vi "QMH Simple Clock Example.vi"() -> ()   [LabVIEW 2013]
uses:
  <userlib>/QMH/examples/Simple Clock/QMH Simple Clock Style.ctl
  <userlib>/QMH/QMH Add Message to Queue (Single Element).vi
  <userlib>/QMH/QMH Add Message to Queue (Array).vi
  <vilib>/Utility/config.llb/Read Key (I32).vi
  <vilib>/Utility/config.llb/Write Key (I32).vi
  <vilib>/Utility/config.llb/NI_LVConfig.lvlib
panel:
  in  "Save State":bool
  out "Seconds":bool[](array[boolean])
  out "Seconds Tens":bool[](array[boolean])
  out "Minutes":bool[](array[boolean])
  out "Minutes Tens":bool[](array[boolean])
  out "Hours":bool[](array[boolean])
  out "Hours Tens":bool[](array[boolean])
  out "Digital":string
  in  "Clock Style":T1
  out "Hour":dbl(knob) scale=0.0..12.0
  out "Minute":dbl(knob) scale=0.0..12.0 scale format="%#.0f"
  out "Status":string
  in  "About":bool
  in  "Exit":bool
  in  "State Variables":cluster{"Config File":path, "Clock Style":T1}
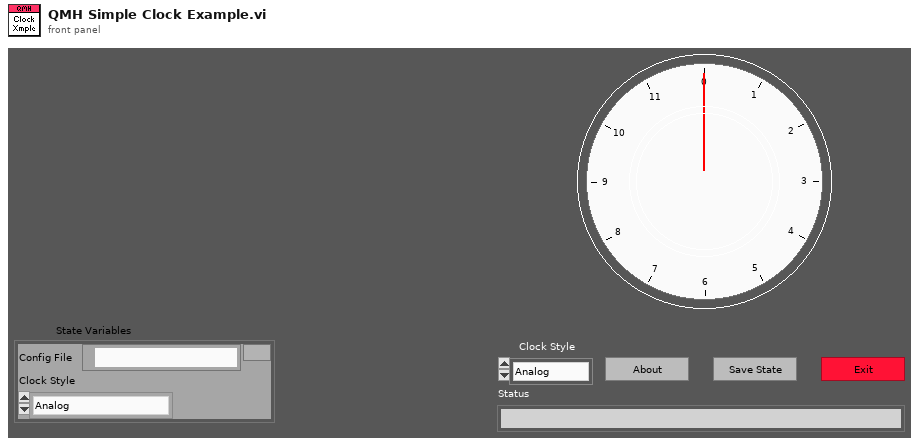
[diagram p1: front panel]
types:
  T1 = typedef "QMH Simple Clock Style.ctl" = enum16{"Analog", "Digital", "Binary"}
  T2 = typedef "LVDateTimeRec.ctl" = cluster{"fractional second":dbl, "second":i32, "minute":i32, "hour":i32, "day of month":i32, "month":i32, "year":i32, "day of week":i32, "day of year":i32, "DST":i32}
  T3 = typedef "NI_LVConfig.lvlib/Config Data RefNum.ctl" = refnum<k1>
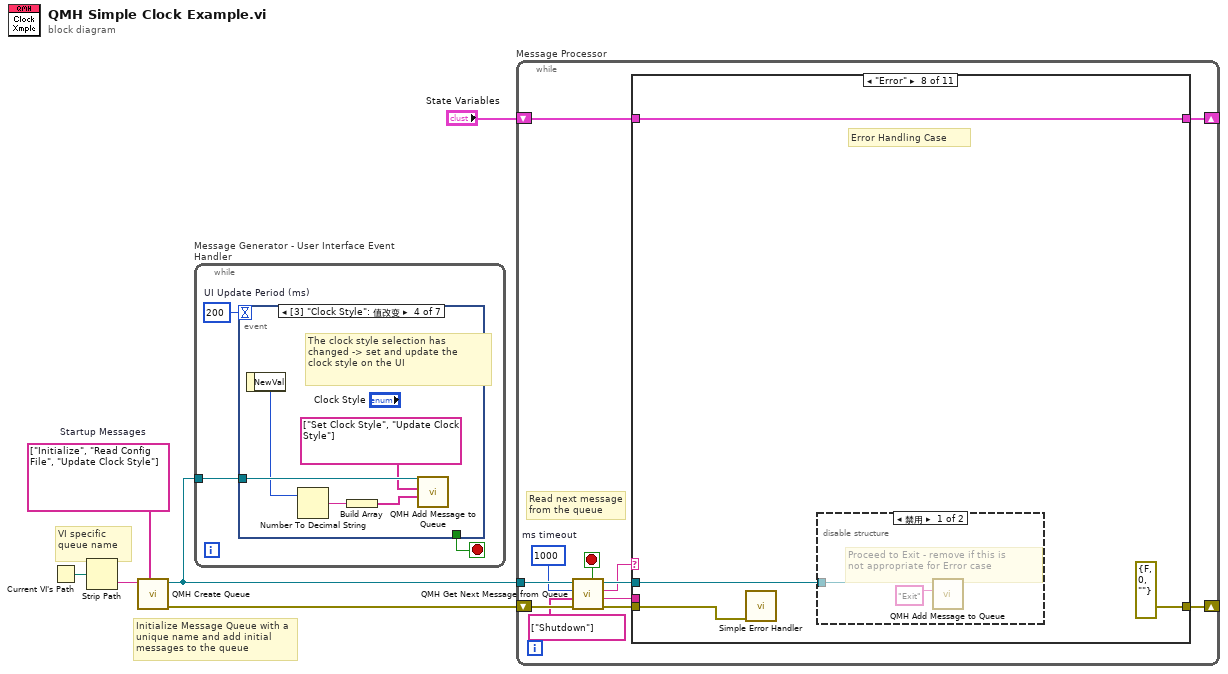
[diagram p0: block diagram]
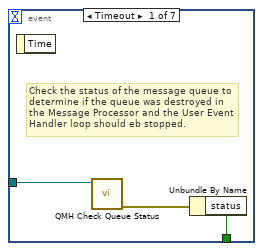
[diagram p2: hidden frame]
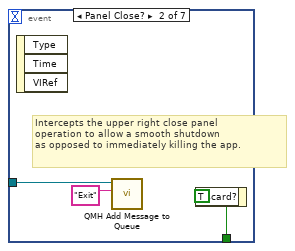
[diagram p3: hidden frame]
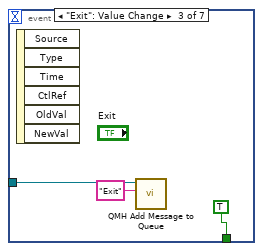
[diagram p4: hidden frame]
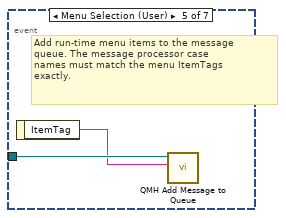
[diagram p5: hidden frame]
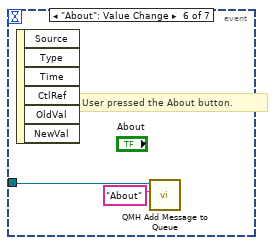
[diagram p6: hidden frame]
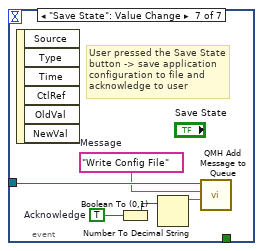
[diagram p7: hidden frame]
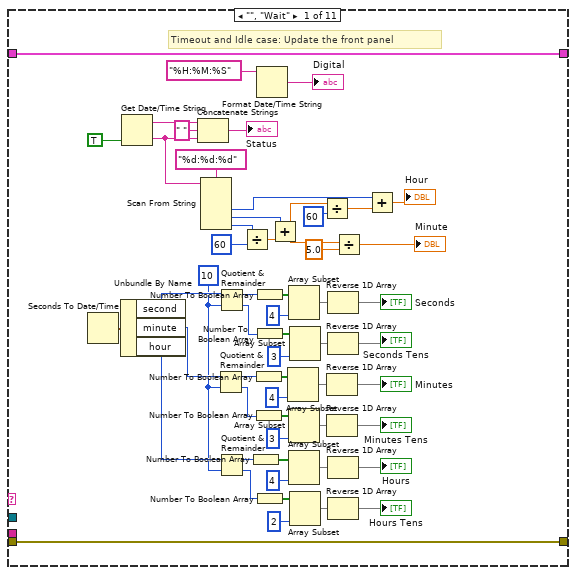
[diagram p8: hidden frame]
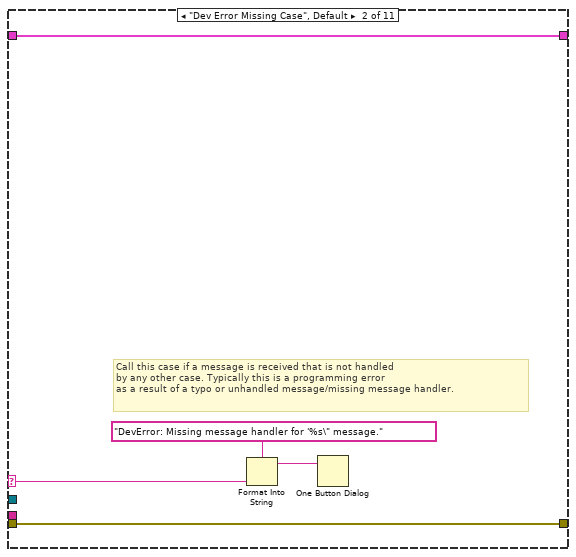
[diagram p9: hidden frame]
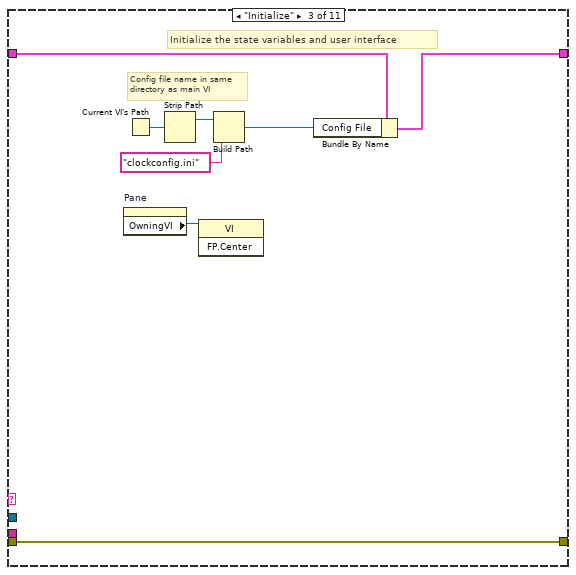
[diagram p10: hidden frame]
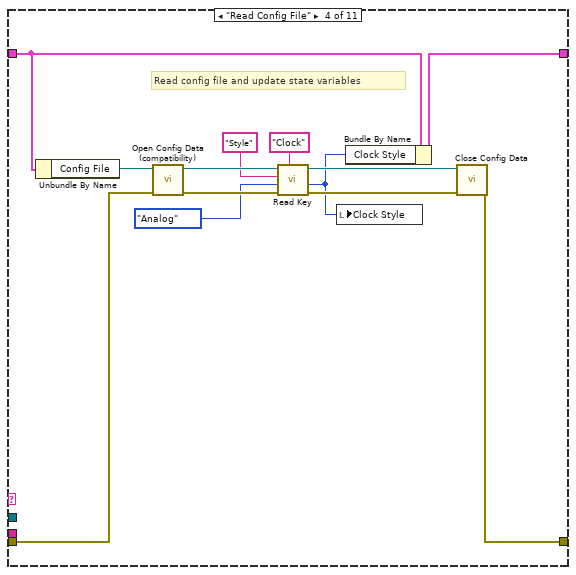
[diagram p11: hidden frame]
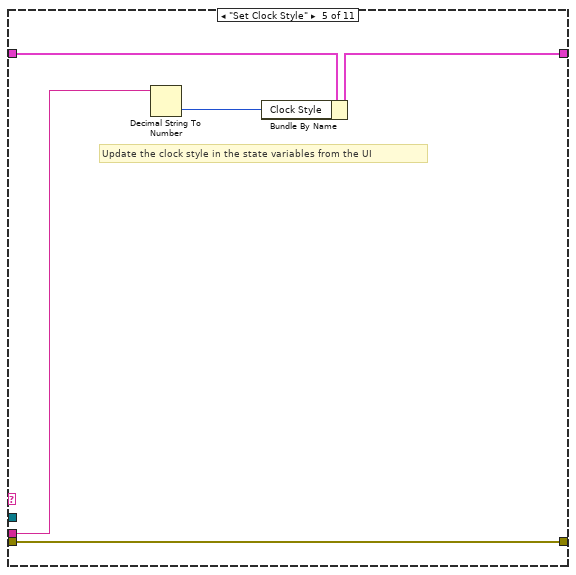
[diagram p12: hidden frame]
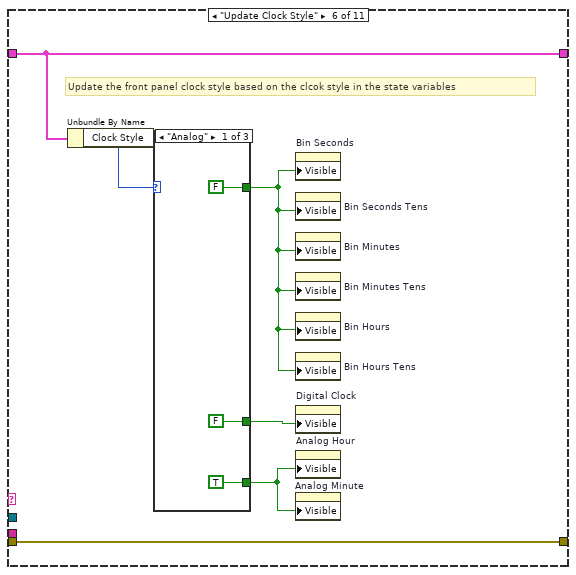
[diagram p13: hidden frame]
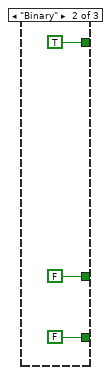
[diagram p14: hidden frame]
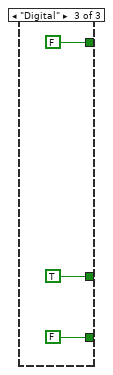
[diagram p15: hidden frame]
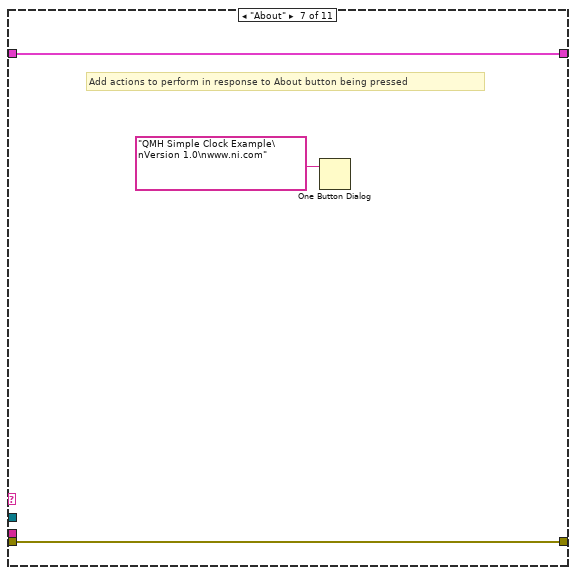
[diagram p16: hidden frame]
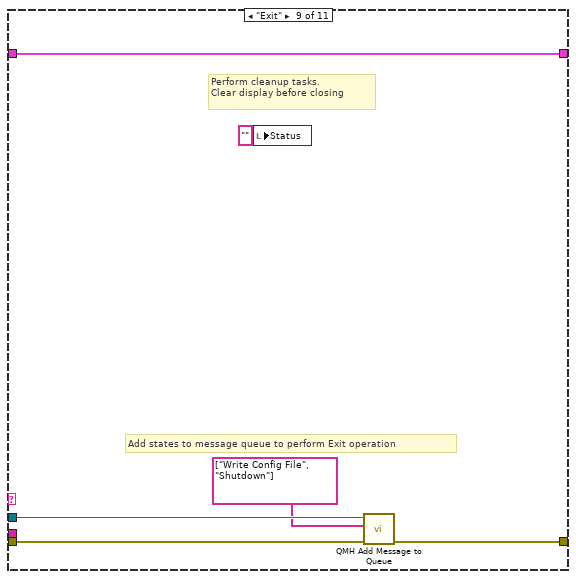
[diagram p18: hidden frame]
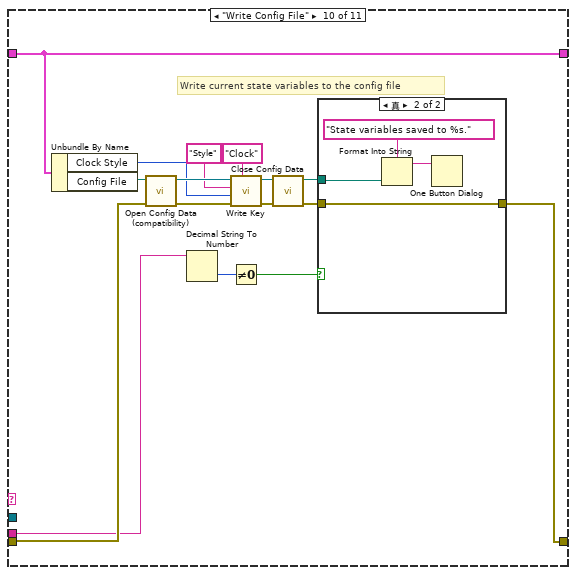
[diagram p19: hidden frame]
diagram:
  w5 = string[] ["Initialize", "Read Config File", "Update Clock Style"]  # Startup Messages
  # "VI specific\nqueue name"
  # "Initialize Message Queue with a unique name and add initial messages to the queue"
  n1 = Current VI's Path() -> (path=w2:path)
  n2 = Strip Path(path=w2) -> (name=w1:string)  [unwired: 1 out]
  n3 = call <userlib>:"QMH Create Queue.vi"("Initial Messages"=w5, "Message queue name (unnamed)"=w1) -> ("error out"=w6:errorcluster, "queue out"=w3:refnum<queue>)  [unwired: 8 in]
  n4 = while "Message Generator - User Interface Event Handler" {
    tunnel: w3 -> [w7]
    stop <- w8 stop-if-true
    w9 = 200  # UI Update Period (ms)
    n5 = event shown="[3] \"Clock Style\": 值改变" {
      selector: _ -> [_ _ _ _ _ _ _]
      dyn-events: _ -> [_ _ _ _ _ _ _]
      timeout: w9 -> [_ _ _ _ _ _ _]
      tunnel: [w12 w15 TRUE ("Discard?") _ _ _ _] -> w8
      tunnel: w7 -> [w11 w14 w17 w23 w25 w27 w32]
      event Timeout {
        # "Check the status of the message queue to determine if the queue was destroyed in the Message Processor and the User Event Handler loop should eb stopped."
        n6 = event-data() -> ()  [unwired: 1 in, 1 out]
        n7 = call <userlib>:"QMH Check Queue Status.vi"("queue in"=w11) -> ("error out"=w10:errorcluster)  [unwired: 7 in, 2 out]
        n8 = Unbundle By Name(w10) -> ("status"=w12:bool)
      }
      event Panel Close? {
        w15 = TRUE ("Discard?")
        # "Intercepts the upper right close panel\noperation to allow a smooth shutdown\nas opposed to immediately killing the app."
        n9 = event-data() -> ()  [unwired: 1 in, 3 out]
        n10 = call-poly <userlib>:"QMH Add Message to Queue.vi"("Message"="Exit", "queue in"=w14) -> ()  [unwired: 8 in, 2 out]
        n11 = event-data("Discard?"=w15) -> ()  [unwired: 1 in, 1 out]
      }
      event "Exit": Value Change {
        n12 = event-data() -> ()  [unwired: 1 in, 6 out]
        n13 = call-poly <userlib>:"QMH Add Message to Queue.vi"("Message"="Exit", "queue in"=w17) -> ()  [unwired: 8 in, 2 out]
      }
      event Value Change {
        # "The clock style selection has\nchanged -> set and update the\nclock style on the UI"
        n14 = event-data() -> ("NewVal"=w19:T1)  [unwired: 1 in]
        n15 = Number To Decimal String(number=w19) -> (decimal integer string=w21:string)  [unwired: 1 in]
        n16 = Build Array(w21) -> (w20:string[])
        n17 = call-poly <userlib>:"QMH Add Message to Queue.vi"("Parameters"=w20, "Messages"=string[] ["Set Clock Style", "Update Clock Style"], "queue in"=w23) -> ()  [unwired: 7 in, 2 out]
      }
      event Menu Selection (User) {
        # "Add run-time menu items to the message\nqueue. The message processor case\nnames must match the menu ItemTags\nexactly."
        n18 = event-data() -> ("ItemTag"=w24:string)  [unwired: 1 in]
        n19 = call-poly <userlib>:"QMH Add Message to Queue.vi"("Message"=w24, "queue in"=w25) -> ()  [unwired: 8 in, 2 out]
      }
      event "About": Value Change {
        # "User pressed the About button."
        n20 = event-data() -> ()  [unwired: 1 in, 6 out]
        n21 = call-poly <userlib>:"QMH Add Message to Queue.vi"("Message"="About", "queue in"=w27) -> ()  [unwired: 8 in, 2 out]
      }
      event "Save State": Value Change {
        w30 = TRUE  # Acknowledge
        w31 = "Write Config File"  # Message
        # "User pressed the Save State button -> save application configuration to file and acknowledge to user"
        n22 = event-data() -> ()  [unwired: 1 in, 6 out]
        n23 = Boolean To (0,1)(Boolean=w30) -> (0, 1=w28:i16)
        n24 = Number To Decimal String(number=w28) -> (decimal integer string=w29:string)  [unwired: 1 in]
        n25 = call-poly <userlib>:"QMH Add Message to Queue.vi"("Parameter"=w29, "Message"=w31, "queue in"=w32) -> ()  [unwired: 7 in, 2 out]
      }
    }
  }
  n26 = while "Message Processor" {
    shift-left: w6 -> [w38]
    shift-right: [w39] -> _
    tunnel: w3 -> [w37]
    shift-left: "State Variables" -> [w44]
    shift-right: [w43] -> _
    stop <- w42 stop-if-true
    w35 = 1000  # ms timeout
    # "Read next message from the queue"
    n27 = call <userlib>:"QMH Get Next Message from Queue.vi"("error in (no error)"=w38, "Termination List ([Exit])"=string[] ["Shutdown"], "ms timeout (1)"=w35, "queue in"=w37) -> ("error out"=w40:errorcluster, "Next Parameter"=w34:string, "Next Message"=w36:string, "queue out"=w41:refnum<queue>, "Stop QMH"=w42:bool)  [unwired: 2 in]
    n28 = case shown="\"Error\"" w36 {
      selector: w36 -> [_ w103 _ _ _ _ _ _ _ _ _]
      tunnel: [w100 w105 w111 w122 w129 w136 w148 w153 w161 w169 w184] -> w43
      tunnel: w44 -> [w100 w105 w112 w118 w130 w136 w148 w153 w161 w169 w184]
      tunnel: w41 -> [_ _ _ _ _ _ _ w150 w159 _ w185]
      tunnel: w40 -> [w99 w104 w113 w116 w131 w137 w149 w151 w158 w168 w186]
      tunnel: [w99 w104 w113 w115 w131 w137 w149 errorcluster {"status"=FALSE, "code"=0, "source"=""} ("error out") w157 w162 w183] -> w39
      tunnel: w34 -> [_ _ _ _ w128 _ _ _ _ w167 _]
      frame "", "Wait" {
        w56 = 10 ("y")
        # "Timeout and Idle case: Update the front panel"
        n29 = Seconds To Date/Time() -> (date time rec=w82:T2)  [unwired: 2 in]
        n30 = Unbundle By Name(w82) -> ("second"=w81:i32, "minute"=w58:i32, "hour"=w57:i32)
        n31 = Get Date/Time String(want seconds? (F)=TRUE) -> (date string=w98:string, time string=w47:string)  [unwired: 2 in]
        n32 = Concatenate Strings(w98, " " ("string"), w47) -> (→"Status":string)
        n33 = Scan From String(format string="%d:%d:%d", input string=w47) -> (output 1=w88:i32, output 2=w91:i32, output 3=w83:i32)  [unwired: 5 in, 3 out]
        n34 = Quotient & Remainder(x=w58, y=w56) -> (x-y*floor(x/y)=w49:i32, floor(x/y)=w65:i32)
        n35 = Quotient & Remainder(x=w81, y=w56) -> (x-y*floor(x/y)=w80:i32, floor(x/y)=w79:i32)
        n36 = Quotient & Remainder(x=w57, y=w56) -> (x-y*floor(x/y)=w54:i32, floor(x/y)=w64:i32)
        n37 = Divide(x=w83, y=60) -> (x/y=w92:dbl)
        n38 = Number To Boolean Array(number=w54) -> (Boolean array=w53:bool[])
        n39 = Number To Boolean Array(number=w49) -> (Boolean array=w48:bool[])
        n40 = Number To Boolean Array(number=w65) -> (Boolean array=w69:bool[])
        n41 = Number To Boolean Array(number=w80) -> (Boolean array=w77:bool[])
        n42 = Number To Boolean Array(number=w79) -> (Boolean array=w74:bool[])
        n43 = Number To Boolean Array(number=w64) -> (Boolean array=w60:bool[])
        n44 = Format Date/Time String(time format string (%c)="%H:%M:%S") -> (date/time string=→"Digital":string)  [unwired: 2 in]
        n45 = Add(x=w91, y=w92) -> (x+y=w86:dbl)
        n46 = Array Subset(array=w48, length=4) -> (w66:bool[])  [unwired: 1 in]
        n47 = Array Subset(array=w77, length=4) -> (w78:bool[])  [unwired: 1 in]
        n48 = Array Subset(array=w69, length=3) -> (w70:bool[])  [unwired: 1 in]
        n49 = Array Subset(array=w53, length=4) -> (w63:bool[])  [unwired: 1 in]
        n50 = Array Subset(array=w74, length=3) -> (w73:bool[])  [unwired: 1 in]
        n51 = Array Subset(array=w60, length=2) -> (w59:bool[])  [unwired: 1 in]
        n52 = Divide(x=w86, y=60) -> (x/y=w89:dbl)
        n53 = Reverse 1D Array(array=w66) -> (reversed array=→"Minutes":bool[])
        n54 = Reverse 1D Array(array=w70) -> (reversed array=→"Minutes Tens":bool[])
        n55 = Reverse 1D Array(array=w78) -> (reversed array=→"Seconds":bool[])
        n56 = Reverse 1D Array(array=w73) -> (reversed array=→"Seconds Tens":bool[])
        n57 = Reverse 1D Array(array=w63) -> (reversed array=→"Hours":bool[])
        n58 = Reverse 1D Array(array=w59) -> (reversed array=→"Hours Tens":bool[])
        n59 = Divide(x=w86, y=5.0) -> (x/y=→"Minute":dbl)
        n60 = Add(x=w88, y=w89) -> (x+y=→"Hour":dbl)
      }
      frame "Dev Error Missing Case", Default {
        # "Call this case if a message is received that is not handled \nby any other case. Typically this is a programming error\nas a result of a typo or unhandled message/missing message handler."
        n61 = Format Into String(format string="DevError: Missing message handler for '%s\" message." ("message"), w103) -> (resulting string=w101:string)  [unwired: 2 in, 1 out]
        n62 = One Button Dialog(message=w101) -> ()  [unwired: 1 in, 1 out]
      }
      frame "Initialize" {
        # "Config file name in same directory as main VI"
        # "Initialize the state variables and user interface"
        n63 = property on="Pane" class="Pane"() -> ("OwningVI"=w106:refnum<vi>)  [unwired: 2 in, 2 out]
        n64 = Current VI's Path() -> (path=w110:path)
        n65 = Strip Path(path=w110) -> (stripped path=w109:path)  [unwired: 1 out]
        n66 = invoke class="VI" method="FP.Center"(reference=w106) -> ()  [unwired: 2 in, 3 out]
        n67 = Build Path(base path=w109, name or relative path="clockconfig.ini") -> (appended path=w107:path)
        n68 = Bundle By Name(cluster=w112, "Config File"=w107) -> (w111:cluster{"Config File":path, "Clock Style":T1})
      }
      frame "Read Config File" {
        # "Read config file and update state variables"
        n69 = Unbundle By Name(w118) -> ("Config File"=w117:path)
        n70 = call <vilib>:"Open Config Data (compatibility).vi"("error in (no error)"=w116, "configuration file path"=w117) -> ("error out"=w126:errorcluster, "refnum"=w125:T3)  [unwired: 7 in, 1 out]
        n71 = call-poly <vilib>:"Read Key.vi"("section"="Clock", "error in (no error)"=w126, "default value"=QMH_Simple_Clock_Style."Analog" ("NewVal"), "key"="Style", "refnum"=w125) -> ("error out"=w119:errorcluster, "value"=w114:i32, "refnum out"=w120:T3)  [unwired: 3 in, 1 out]
        n72 = local write "Clock Style"(w114) -> ()
        n73 = Bundle By Name(cluster=w118, "Clock Style"=w114) -> (w122:cluster{"Config File":path, "Clock Style":T1})
        n74 = call <vilib>:"Close Config Data.vi"("error in (no error)"=w119, "refnum"=w120) -> ("error out"=w115:errorcluster)  [unwired: 8 in, 1 out]
      }
      frame "Set Clock Style" {
        # "Update the clock style in the state variables from the UI"
        n75 = Decimal String To Number(string=w128) -> (number=w127:i32)  [unwired: 2 in, 1 out]
        n76 = Bundle By Name(cluster=w130, "Clock Style"=w127) -> (w129:cluster{"Config File":path, "Clock Style":T1})
      }
      frame "Update Clock Style" {
        # "Update the front panel clock style based on the clcok style in the state variables"
        n77 = Unbundle By Name(w136) -> ("Clock Style"=w135:T1)
        n78 = case shown="\"Analog\"" w135 {
          tunnel: [FALSE FALSE TRUE] -> w134
          tunnel: [TRUE FALSE FALSE] -> w133
          tunnel: [FALSE TRUE FALSE] -> w132
          frame "Analog" {
          }
          frame "Binary" {
          }
          frame "Digital" {
          }
        }
        n79 = property on="Bin Seconds" class="Arr (严格)"("Visible"=w132) -> ()  [unwired: 2 in, 2 out]
        n80 = property on="Bin Seconds Tens" class="Arr (严格)"("Visible"=w132) -> ()  [unwired: 2 in, 2 out]
        n81 = property on="Bin Minutes" class="Arr (严格)"("Visible"=w132) -> ()  [unwired: 2 in, 2 out]
        n82 = property on="Bin Minutes Tens" class="Arr (严格)"("Visible"=w132) -> ()  [unwired: 2 in, 2 out]
        n83 = property on="Bin Hours" class="Arr (严格)"("Visible"=w132) -> ()  [unwired: 2 in, 2 out]
        n84 = property on="Bin Hours Tens" class="Arr (严格)"("Visible"=w132) -> ()  [unwired: 2 in, 2 out]
        n85 = property on="Digital Clock" class="Str"("Visible"=w134) -> ()  [unwired: 2 in, 2 out]
        n86 = property on="Analog Hour" class="Knob (严格)"("Visible"=w133) -> ()  [unwired: 2 in, 2 out]
        n87 = property on="Analog Minute" class="Knob (严格)"("Visible"=w133) -> ()  [unwired: 2 in, 2 out]
      }
      frame "About" {
        # "Add actions to perform in response to About button being pressed"
        n88 = One Button Dialog(message="QMH Simple Clock Example\nVersion 1.0\nwww.ni.com") -> ()  [unwired: 1 in, 1 out]
      }
      frame "Error" {
        # "Error Handling Case"
        n89 = call <vilib>:"Simple Error Handler.vi"("error in (no error)"=w151) -> ()  [unwired: 4 in, 5 out]
        n90 = disable-structure shown="禁用" {
          disable-tunnel: w150 -> [w155 _]
          frame Disabled {
            # "Proceed to Exit - remove if this is\nnot appropriate for Error case"
            n91 = call-poly <userlib>:"QMH Add Message to Queue.vi"("Message"="Exit", "queue in"=w155) -> ()  [unwired: 8 in, 2 out]
          }
          frame Enabled {
          }
        }
      }
      frame "Exit" {
        # "Add states to message queue to perform Exit operation"
        # "Perform cleanup tasks.\nClear display before closing"
        n92 = local write "Status"("" ("Status")) -> ()
        n93 = call-poly <userlib>:"QMH Add Message to Queue.vi"("error in (no error)"=w158, "Messages"=string[] ["Write Config File", "Shutdown"], "queue in"=w159) -> ("error out"=w157:errorcluster)  [unwired: 7 in, 1 out]
      }
      frame "Write Config File" {
        # "Write current state variables to the config file"
        n94 = Unbundle By Name(w169) -> ("Clock Style"=w170:T1, "Config File"=w171:path)
        n95 = call <vilib>:"Open Config Data (compatibility).vi"("error in (no error)"=w168, "configuration file path"=w171) -> ("error out"=w177:errorcluster, "refnum"=w176:T3)  [unwired: 7 in, 1 out]
        n96 = Decimal String To Number(string=w167) -> (number=w166:i32)  [unwired: 2 in, 1 out]
        n97 = call-poly <vilib>:"Write Key.vi"("section"="Clock", "error in (no error)"=w177, "value"=w170, "key"="Style", "refnum"=w176) -> ("error out"=w172:errorcluster, "refnum out"=w173:T3)  [unwired: 4 in, 1 out]
        n98 = Not Equal To 0?(x=w166) -> (x != 0?=w165:bool)
        n99 = call <vilib>:"Close Config Data.vi"("error in (no error)"=w172, "refnum"=w173) -> ("error out"=w164:errorcluster, "file path"=w163:path)  [unwired: 8 in]
        n100 = case shown="真" w165 {
          tunnel: w164 -> [w178 w179]
          tunnel: w163 -> [_ w182]
          tunnel: [w178 w179] -> w162
          frame False {
          }
          frame True {
            n101 = Format Into String(format string="State variables saved to %s.", w182) -> (resulting string=w180:string)  [unwired: 2 in, 1 out]
            n102 = One Button Dialog(message=w180) -> ()  [unwired: 1 in, 1 out]
          }
        }
      }
      frame "Shutdown" {
        n103 = call <userlib>:"QMH Destroy Queue.vi"("error in (no error)"=w186, "queue in"=w185) -> ("error out"=w183:errorcluster)  [unwired: 7 in, 2 out]
      }
    }
  }
